vi "Table Set Value To Selection.vi"(8 "error in":errorcluster, 9 "String":string, 11 "Table Ref In":refnum<vi>) -> (0 "error out":errorcluster, 3 "Table Ref Out":refnum<vi>)   [LabVIEW 2024]
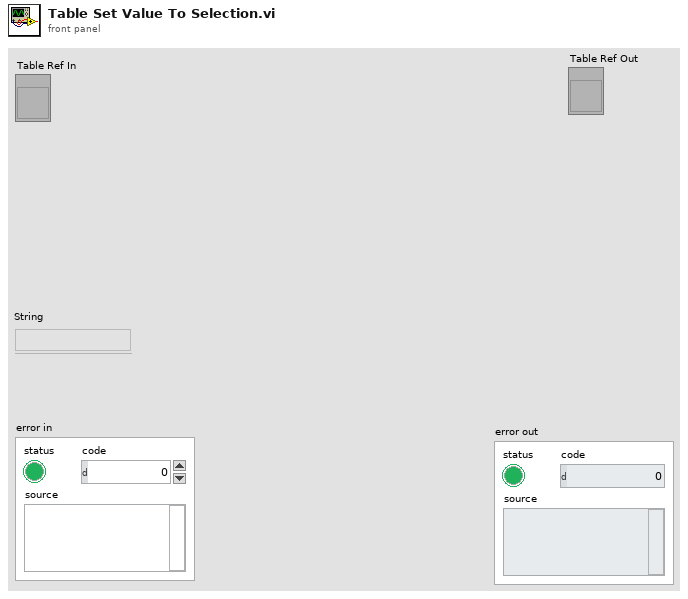
[diagram p1: front panel]
types:
  T1 = typedef "LVRowAndColumnTypeDef.ctl" = cluster{"Row":i32, "Column":i32}
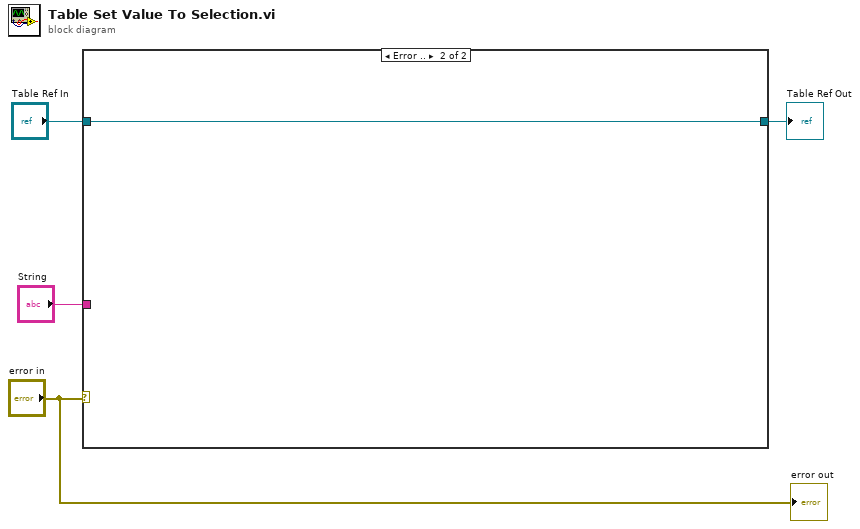
[diagram p0: block diagram]
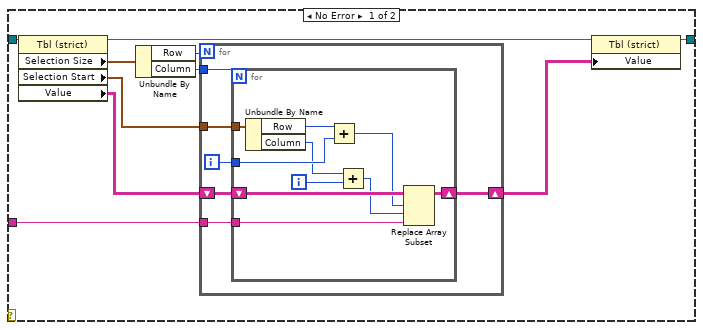
[diagram p2: hidden frame]
diagram:
  n1 = case shown="Error .." "error in" {
    tunnel: "Table Ref In" -> [w13 w31]
    tunnel: [w12 w31] -> w3
    tunnel: "String" -> [w6 _]
    frame No Error {
      n2 = property class="Tbl (strict)"(reference=w13) -> (reference out=w14:refnum<vi>, "Selection Size"=w11:T1, "Selection Start"=w8:T1, "Value"=w7:string[][])  [unwired: 1 in, 1 out]
      n3 = Unbundle By Name(w11) -> ("Row"=w10:i32, "Column"=w9:i32)
      n4 = for {
        N: w10 -> [_]
        tunnel: w9 -> [w20]
        tunnel: w8 -> [w19]
        shift-right: [w16] -> w5
        shift-left: w7 -> [w18]
        tunnel: w6 -> [w17]
        i -> [w15]
        n5 = for {
          N: w20 -> [_]
          tunnel: w19 -> [w28]
          shift-right: [w29] -> w16
          shift-left: w18 -> [w30]
          tunnel: w17 -> [w21]
          tunnel: w15 -> [w26]
          i -> [w23]
          n6 = Unbundle By Name(w28) -> ("Row"=w27:i32, "Column"=w24:i32)
          n7 = Add(x=w27, y=w26) -> (x+y=w25:i32)
          n8 = Add(x=w24, y=w23) -> (x+y=w22:i32)
          n9 = Replace Array Subset(array=w30, new element=w21, index (row)=w25, index (col)=w22) -> (w29:string[][])
        }
      }
      n10 = property class="Tbl (strict)"(reference=w14, "Value"=w5) -> (reference out=w12:refnum<vi>)  [unwired: 1 in, 1 out]
    }
    frame Error {
    }
  }
  "Table Ref Out" <- w3
  "error out" <- "error in"
